vi "Calc Moments.vi"(9 "Calibration":dbl[unit]=0.0002667495458183679, 11 "image array":dbl[][](array[numeric])) -> (0 "Durchmesser Y":dbl[unit]=0.00021926520750996826, 1 "Durchmesser X":dbl[unit]=0.00023644934901996347, 2 "2nd Moment y":dbl[unit]=1.3977073662991126e-08, 3 "2nd Moment x":dbl[unit]=1.2019307806097362e-08, 5 "1st Moment y":dbl[unit]=0.00022599485342451785, 7 "1st Moment x":dbl[unit]=0.0002667495458183679)   [LabVIEW 2014, in "Analyze.lvlib" / "Analyze SecondMomentum.lvclass"]
uses:
  Analyze SecondMomentum.lvclass
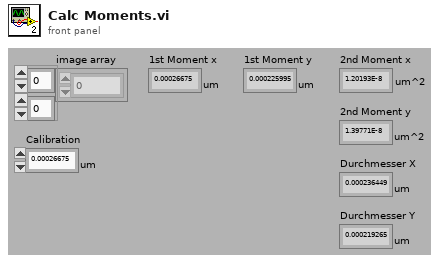
[diagram p1: front panel]
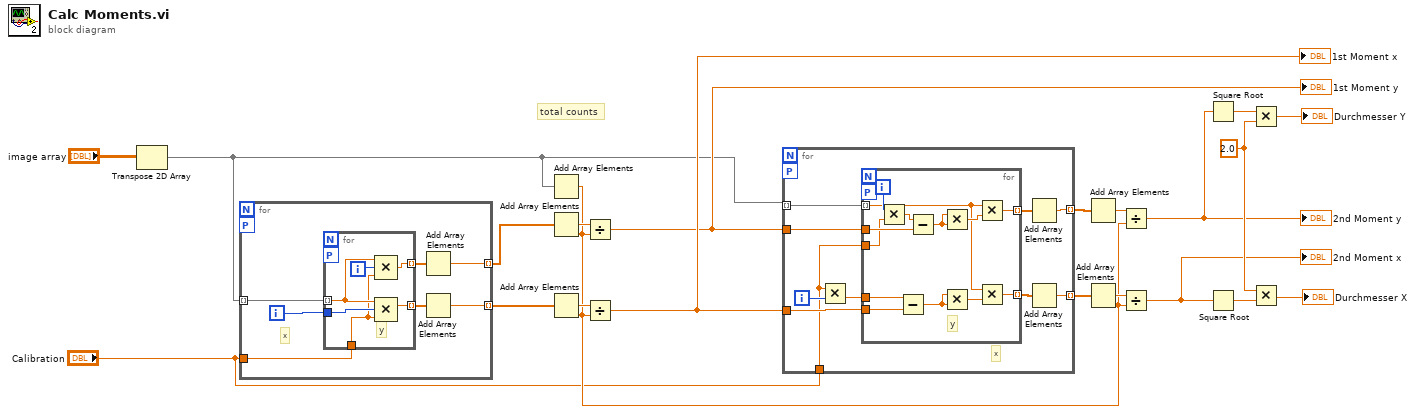
[diagram p0: block diagram]
diagram:
  w8 = 2.0 ("x")
  # "total counts"
  n1 = Transpose 2D Array(2D array="image array") -> (transposed array=w4:dbl[][])
  n2 = for {
    tunnel: w4 -> [w28] mode=indexing
    tunnel: [w22] -> w21 mode=indexing
    tunnel: [w24] -> w19 mode=indexing
    tunnel: "Calibration" -> [w23]
    workers-P: _ -> [_]
    i -> [w26]
    # "x"
    n3 = for {
      tunnel: w28 -> [w32] mode=indexing
      tunnel: [w33] -> w27 mode=indexing
      tunnel: w26 -> [w31]
      tunnel: [w30] -> w25 mode=indexing
      tunnel: w23 -> [w29]
      workers-P: _ -> [_]
      i -> [w34]
      # "y"
      n4 = Compound Arithmetic op=MULTIPLY(w32, w34, w29) -> (w33:dbl[unit])
      n5 = Compound Arithmetic op=MULTIPLY(w32, w31, w29) -> (w30:dbl[unit])
    }
    n6 = Add Array Elements(numeric array=w27) -> (sum=w22:dbl[unit])
    n7 = Add Array Elements(numeric array=w25) -> (sum=w24:dbl[unit])
  }
  n8 = Add Array Elements(numeric array=w4) -> (sum=w11:dbl)
  n9 = Add Array Elements(numeric array=w21) -> (sum=w20:dbl[unit])
  n10 = Add Array Elements(numeric array=w19) -> (sum=w18:dbl[unit])
  n11 = Divide(x=w20, y=w11) -> (x/y=w15:dbl[unit])
  "1st Moment y" <- w15
  n12 = Divide(x=w18, y=w11) -> (x/y=w17:dbl[unit])
  "1st Moment x" <- w17
  n13 = for {
    tunnel: w4 -> [w44] mode=indexing
    tunnel: w17 -> [w42]
    tunnel: [w40] -> w16 mode=indexing
    tunnel: w15 -> [w39]
    tunnel: [w37] -> w14 mode=indexing
    tunnel: "Calibration" -> [w35]
    workers-P: _ -> [_]
    i -> [w43]
    # "x"
    n14 = Multiply(x=w35, y=w43) -> (x*y=w36:dbl[unit])
    n15 = for {
      tunnel: w44 -> [w48] mode=indexing
      tunnel: w36 -> [w57]
      tunnel: w42 -> [w56]
      tunnel: [w53] -> w41 mode=indexing
      tunnel: w39 -> [w51]
      tunnel: [w47] -> w38 mode=indexing
      tunnel: w35 -> [w45]
      workers-P: _ -> [_]
      i -> [w52]
      # "y"
      n16 = Multiply(x=w52, y=w45) -> (x*y=w46:dbl[unit])
      n17 = Subtract(x=w57, y=w56) -> (x-y=w55:dbl[unit])
      n18 = Subtract(x=w46, y=w51) -> (x-y=w50:dbl[unit])
      n19 = Multiply(x=w50, y=w50) -> (x*y=w49:dbl[unit])
      n20 = Multiply(x=w55, y=w55) -> (x*y=w54:dbl[unit])
      n21 = Multiply(x=w48, y=w49) -> (x*y=w47:dbl[unit])
      n22 = Multiply(x=w48, y=w54) -> (x*y=w53:dbl[unit])
    }
    n23 = Add Array Elements(numeric array=w38) -> (sum=w37:dbl[unit])
    n24 = Add Array Elements(numeric array=w41) -> (sum=w40:dbl[unit])
  }
  n25 = Add Array Elements(numeric array=w14) -> (sum=w12:dbl[unit])
  n26 = Add Array Elements(numeric array=w16) -> (sum=w13:dbl[unit])
  n27 = Divide(x=w12, y=w11) -> (x/y=w2:dbl[unit])
  "2nd Moment y" <- w2
  n28 = Divide(x=w13, y=w11) -> (x/y=w1:dbl[unit])
  "2nd Moment x" <- w1
  n29 = Square Root(x=w2) -> (sqrt(x)=w10:dbl[unit])
  n30 = Square Root(x=w1) -> (sqrt(x)=w9:dbl[unit])
  n31 = Multiply(x=w10, y=w8) -> (x*y=→"Durchmesser Y":dbl[unit])
  n32 = Multiply(x=w8, y=w9) -> (x*y=→"Durchmesser X":dbl[unit])
